vi "Close VI Reference.vi"(8 "error in (no error)":errorcluster, 11 "VI Reference":refnum<vi>) -> (0 "error out":errorcluster)   [LabVIEW 2010]
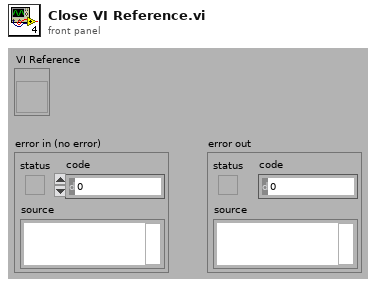
[diagram p1: front panel]
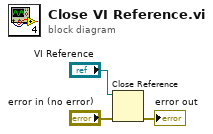
[diagram p0: block diagram]
diagram:
  n1 = Close Reference(reference="VI Reference", error in (no error)="error in (no error)") -> (error out=→"error out":errorcluster)
